vi "PWM Command_TS.vi"(8 "error in (no error) 2":errorcluster, 9 "Leg":i32 min=0 max=6, 10 "Duty Cycle":i32 min=0 max=100) -> (0 "error out":errorcluster, 1 "return count":u32, 3 "VISA Refnum out":refnum<visa-resource-name>, 4 "read buffer":string, 5 "Set PWM Leg":string, 6 "Set Duty Cycle":string, 7 ">":string, 11 "Duty Cycle VISA Write":string)   [LabVIEW 2022 SP3]
uses:
  <vilib>/Instr/_visa.llb/VISA Configure Serial Port (Instr).vi
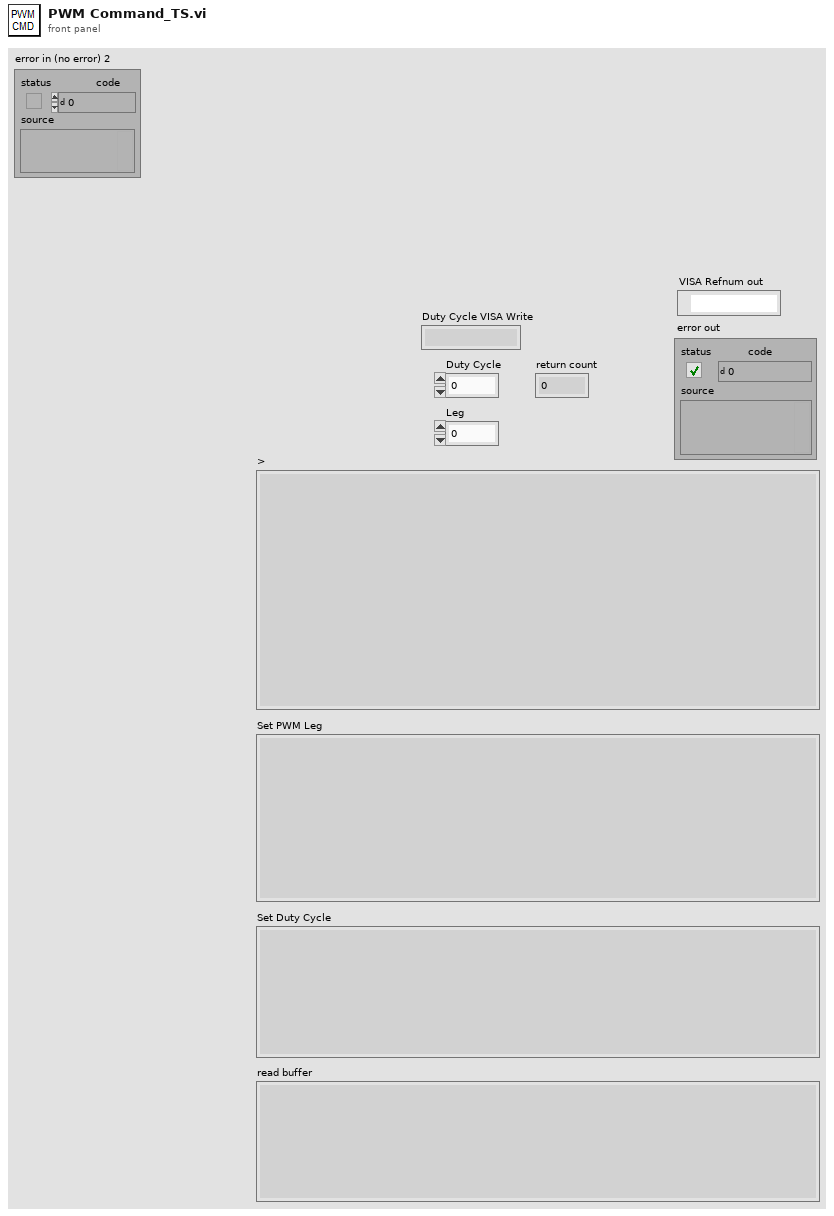
[diagram p1: front panel]
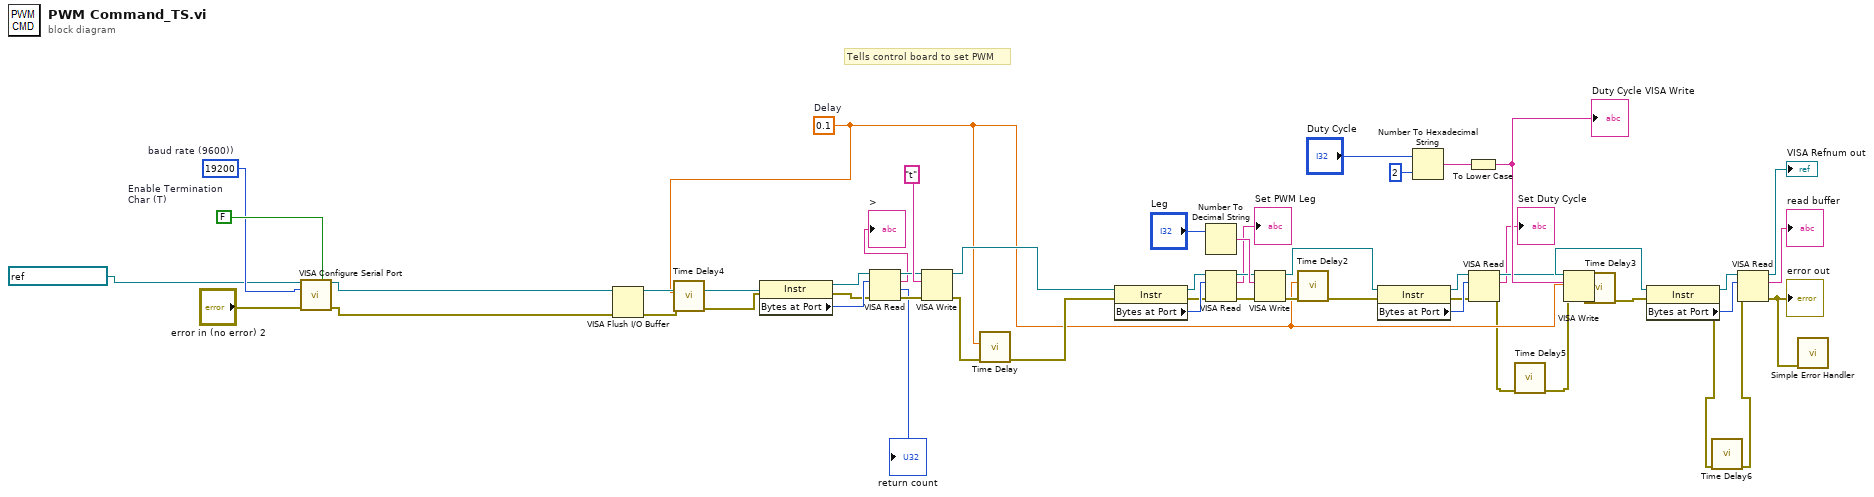
[diagram p0: block diagram]
diagram:
  w5 = u32 19200  # baud rate (9600))
  w6 = FALSE  # Enable Termination Char (T)
  w11 = 0.1  # Delay
  # "Tells control board to set PWM"
  n1 = call-poly "VISA Configure Serial Port"("VISA resource name"=refnum<visa-resource-name> "ControlBoard", "Enable Termination\nChar (T)"=w6, "baud rate (9600)"=w5, "error in (no error)"="error in (no error) 2") -> ("VISA resource name out"=w3:refnum<visa-resource-name>, "error out"=w2:errorcluster)  [unwired: 10 in]
  n2 = VISA Flush I/O Buffer(VISA resource name=w3, error in (no error)=w2) -> (VISA resource name out=w14:refnum<visa-resource-name>, error out=w13:errorcluster)  [unwired: 1 in]
  n3 = call "Time Delay4"("error in (no error)"=w13, "Delay Time (s)"=w11) -> ("error out"=w12:errorcluster)  [unwired: 9 in]
  n4 = property class="Instr"(reference=w14, error in=w12) -> (reference out=w34:refnum<visa-resource-name>, error out=w16:errorcluster, "Bytes at Port"=w33:u32)
  n5 = VISA Read(VISA resource name=w34, byte count=w33, error in (no error)=w16) -> (VISA resource name out=w35:refnum<visa-resource-name>, read buffer=→">":string, return count=→"return count":u32, error out=w36:errorcluster)
  n6 = VISA Write(VISA resource name=w35, write buffer="t", error in (no error)=w36) -> (VISA resource name out=w48:refnum<visa-resource-name>, error out=w53:errorcluster)  [unwired: 1 out]
  n7 = call "Time Delay"("error in (no error)"=w53, "Delay Time (s)"=w11) -> ("error out"=w31:errorcluster)  [unwired: 9 in]
  n8 = property class="Instr"(reference=w48, error in=w31) -> (reference out=w39:refnum<visa-resource-name>, error out=w30:errorcluster, "Bytes at Port"=w38:u32)
  n9 = Number To Decimal String(number="Leg") -> (decimal integer string=w42:string)  [unwired: 1 in]
  n10 = VISA Read(VISA resource name=w39, byte count=w38, error in (no error)=w30) -> (VISA resource name out=w41:refnum<visa-resource-name>, read buffer=→"Set PWM Leg":string, error out=w40:errorcluster)  [unwired: 1 out]
  n11 = VISA Write(VISA resource name=w41, write buffer=w42, error in (no error)=w40) -> (VISA resource name out=w47:refnum<visa-resource-name>, error out=w46:errorcluster)  [unwired: 1 out]
  n12 = call "Time Delay2"("error in (no error)"=w46, "Delay Time (s)"=w11) -> ("error out"=w24:errorcluster)  [unwired: 9 in]
  n13 = property class="Instr"(reference=w47, error in=w24) -> (reference out=w28:refnum<visa-resource-name>, error out=w25:errorcluster, "Bytes at Port"=w27:u32)
  n14 = Number To Hexadecimal String(1:i16 2 ("width (-)"), 2:"Duty Cycle") -> (0:w50:string)
  n15 = To Lower Case(string=w50) -> (all lower case string=w49:string)
  "Duty Cycle VISA Write" <- w49
  n16 = VISA Read(VISA resource name=w28, byte count=w27, error in (no error)=w25) -> (VISA resource name out=w29:refnum<visa-resource-name>, read buffer=→"Set Duty Cycle":string, error out=w10:errorcluster)  [unwired: 1 out]
  n17 = call "Time Delay5"("error in (no error)"=w10) -> ("error out"=w9:errorcluster)  [unwired: 10 in]
  n18 = VISA Write(VISA resource name=w29, write buffer=w49, error in (no error)=w9) -> (VISA resource name out=w51:refnum<visa-resource-name>, error out=w45:errorcluster)  [unwired: 1 out]
  n19 = call "Time Delay3"("error in (no error)"=w45, "Delay Time (s)"=w11) -> ("error out"=w19:errorcluster)  [unwired: 9 in]
  n20 = property class="Instr"(reference=w51, error in=w19) -> (reference out=w22:refnum<visa-resource-name>, error out=w8:errorcluster, "Bytes at Port"=w21:u32)
  n21 = call "Time Delay6"("error in (no error)"=w8) -> ("error out"=w7:errorcluster)  [unwired: 10 in]
  n22 = VISA Read(VISA resource name=w22, byte count=w21, error in (no error)=w7) -> (VISA resource name out=→"VISA Refnum out":refnum<visa-resource-name>, read buffer=→"read buffer":string, error out=w17:errorcluster)  [unwired: 1 out]
  "error out" <- w17
  n23 = call <vilib>:"Simple Error Handler.vi"("error in (no error)"=w17) -> ()  [unwired: 4 in, 5 out]
